vi "Untitled 19 (SubVI).vi"(9 "Fuel type":bool, 10 "Stoic condition":dbl, 11 "T02":dbl) -> (3 "T03":dbl)   [LabVIEW 2019]
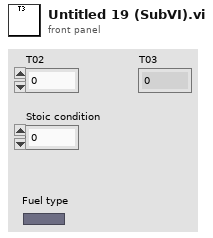
[diagram p1: front panel]
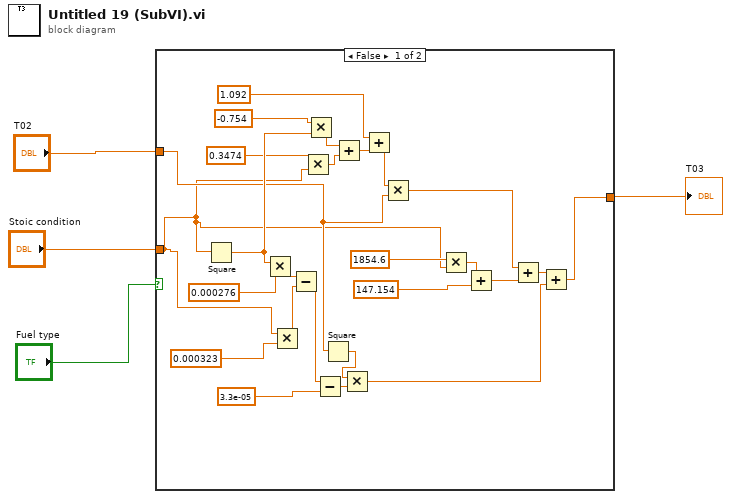
[diagram p0: block diagram]
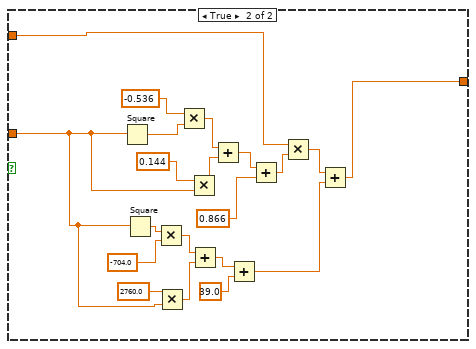
[diagram p2: hidden frame]
diagram:
  n1 = case shown="False" "Fuel type" {
    tunnel: [w5 w50] -> w4
    tunnel: "Stoic condition" -> [w6 w45]
    tunnel: "T02" -> [w16 w39]
    frame False {
      n2 = Square(x=w6) -> (x^2=w22:dbl)
      n3 = Multiply(x=w22, y=0.000276) -> (x*y=w29:dbl)
      n4 = Multiply(x=w6, y=0.000323) -> (x*y=w27:dbl)
      n5 = Subtract(x=w29, y=w27) -> (x-y=w26:dbl)
      n6 = Multiply(x=0.3474, y=w6) -> (x*y=w20:dbl)
      n7 = Multiply(x=-0.754, y=w22) -> (x*y=w19:dbl)
      n8 = Subtract(x=w26, y=3.3e-05) -> (x-y=w9:dbl)
      n9 = Square(x=w16) -> (x^2=w24:dbl)
      n10 = Add(x=w19, y=w20) -> (x+y=w18:dbl)
      n11 = Multiply(x=w24, y=w9) -> (x*y=w11:dbl)
      n12 = Add(x=1.092, y=w18) -> (x+y=w8:dbl)
      n13 = Multiply(x=w8, y=w16) -> (x*y=w10:dbl)
      n14 = Multiply(x=1854.6, y=w6) -> (x*y=w14:dbl)
      n15 = Add(x=w14, y=147.154) -> (x+y=w7:dbl)
      n16 = Add(x=w10, y=w7) -> (x+y=w12:dbl)
      n17 = Add(x=w12, y=w11) -> (x+y=w5:dbl)
    }
    frame True {
      n18 = Square(x=w45) -> (x^2=w31:dbl)
      n19 = Square(x=w45) -> (x^2=w41:dbl)
      n20 = Multiply(x=w41, y=-704.0) -> (x*y=w43:dbl)
      n21 = Multiply(x=2760.0, y=w45) -> (x*y=w46:dbl)
      n22 = Multiply(x=-0.536, y=w31) -> (x*y=w33:dbl)
      n23 = Multiply(x=0.144, y=w45) -> (x*y=w34:dbl)
      n24 = Add(x=w43, y=w46) -> (x+y=w47:dbl)
      n25 = Add(x=w33, y=w34) -> (x+y=w36:dbl)
      n26 = Add(x=w47, y=39.0) -> (x+y=w49:dbl)
      n27 = Add(x=w36, y=0.866) -> (x+y=w38:dbl)
      n28 = Multiply(x=w39, y=w38) -> (x*y=w40:dbl)
      n29 = Add(x=w40, y=w49) -> (x+y=w50:dbl)
    }
  }
  "T03" <- w4
